vi "Parse State Queue Plus.vi"(0 "State Queue":string, 1 "Name(\"\" to use uuid)":string, 7 "Error In (no error)":errorcluster, 9 "Dequeue Timeout(0ms)":i32, 11 "Response Timeout(1000ms)":i32=1000) -> (4 "Remaining States":string, 6 "Current State":string, 8 "Arguments":string, 15 "From Who":string)   [LabVIEW 2020, in "JKI-State-Machine-Plus.lvlib"]
doc: "Parses the JKI State Machine state queue and returns the current state that will execute next with the associated arguments.\n\nFor instructions on how to use the JKI State Machine, examples and video tutorials, visit:\nhttp://jkisoft.com/state-machine/\n\n<B>Inputs:</B>\n <B>State Queue:</B> The entire state queue is wired to this input. This should come from the main JKI State Machine shift register.\n <B>Error In</B> The error cluster from the JKI State Machine is wired to this input. If an error occures and appears on this input, the current state output returns the \"Error Handler\" state.\n\n<B>Outputs:</B>\n <B>Remaining States:</B> Returns all the next states that should execute after the current state completes. These should be passed through the current state in the state machine. These can also be modified or augmented within the current state if necessary.\n <B>Current State:</B> Returns the current state that should execute next in the state machine. If an error is wired to the Error input then the current state output becomes \"Error Handler\".\n <B>Arguments:</B> Returns any argument(s) that may be used in the current state string. These arguments come after the \">>\" characters. <B>Note:</B> The arguments variable must not contain any unprintable characters like linefeed or carriage return.\n\n<B>State Syntax:</B>\nStateCategory: State >> Argument\nLine Terminator: Line feed\n <B>Example:</B>\nUI: Help >> About\n\nWhere \"UI\" is the state category\nWhere \"Help\" is the state\nWhere \"About\" is the argument\n <B>Other Examples:</B>\nApp Data: Initialize\nUI: Initialize\nHelp >> About\n\n<B>Commenting:</B>\nTo add a comment use \"//\" or \"#\" and all text to the right will be ignored\n <B>Commenting Example:</B>\nUI: Initialize // This initializes the UI\n# This whole line is a comment\n// Another comment line\n\nJKI State Machine™ 2018.0.7.45\nhttp://jki.net/state-machine/\nCopyright (C) 2005-2018, JKI <info@jki.net>\nALL RIGHTS RESERVED"
uses:
  JKI-State-Machine-Plus.lvlib
  _Cross JKI StateMachine State Data.ctl
  _Cross JKI StateMachine State Response.ctl
  _uuid.vi
  _JKISMQFGV.vi
  <vilib>/regexp/Match Regular Expression.xnode
panel:
  # "For instructions on how to use the JKI State Machine, examples and video tutorials, visit:\nhttp://jki.net/state-machine/\n\nJKI State Machine™\nhttp://jki.net/state-machine/\nCopyright (C) 2005-2017, JKI <info@jki.net>\nALL RIGHTS RESERVED"
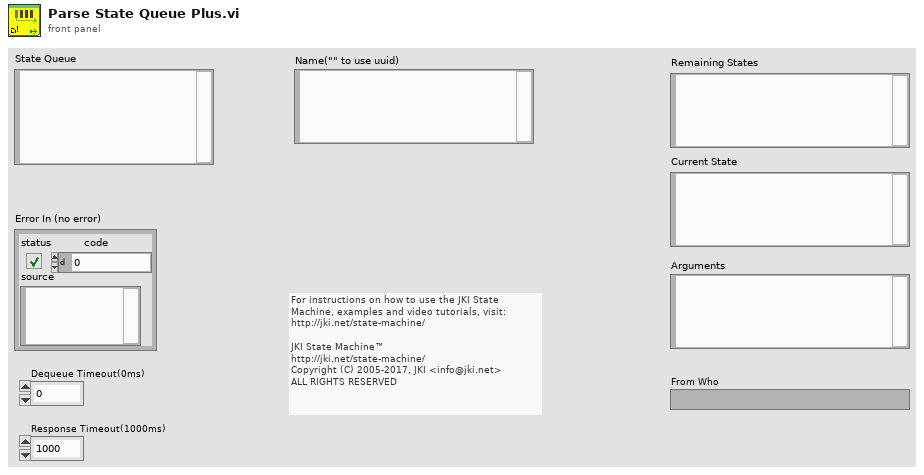
[diagram p1: front panel]
types:
  T1 = typedef "JKI-State-Machine-Plus.lvlib/_Cross JKI StateMachine State Data.ctl" = cluster{"state":string, "args":string, "source":string, "RespQ":refnum<queue>}
  T2 = typedef "JKI-State-Machine-Plus.lvlib/_Cross JKI StateMachine State Response.ctl" = cluster{"error":errorcluster}
  T3 = typedef "JKI-State-Machine-Plus.lvlib/_JKISMQ.ctl" = cluster{"Queue":refnum<queue>, "Locked Status":refnum<data-value>, "Stand Alone Mode":bool}
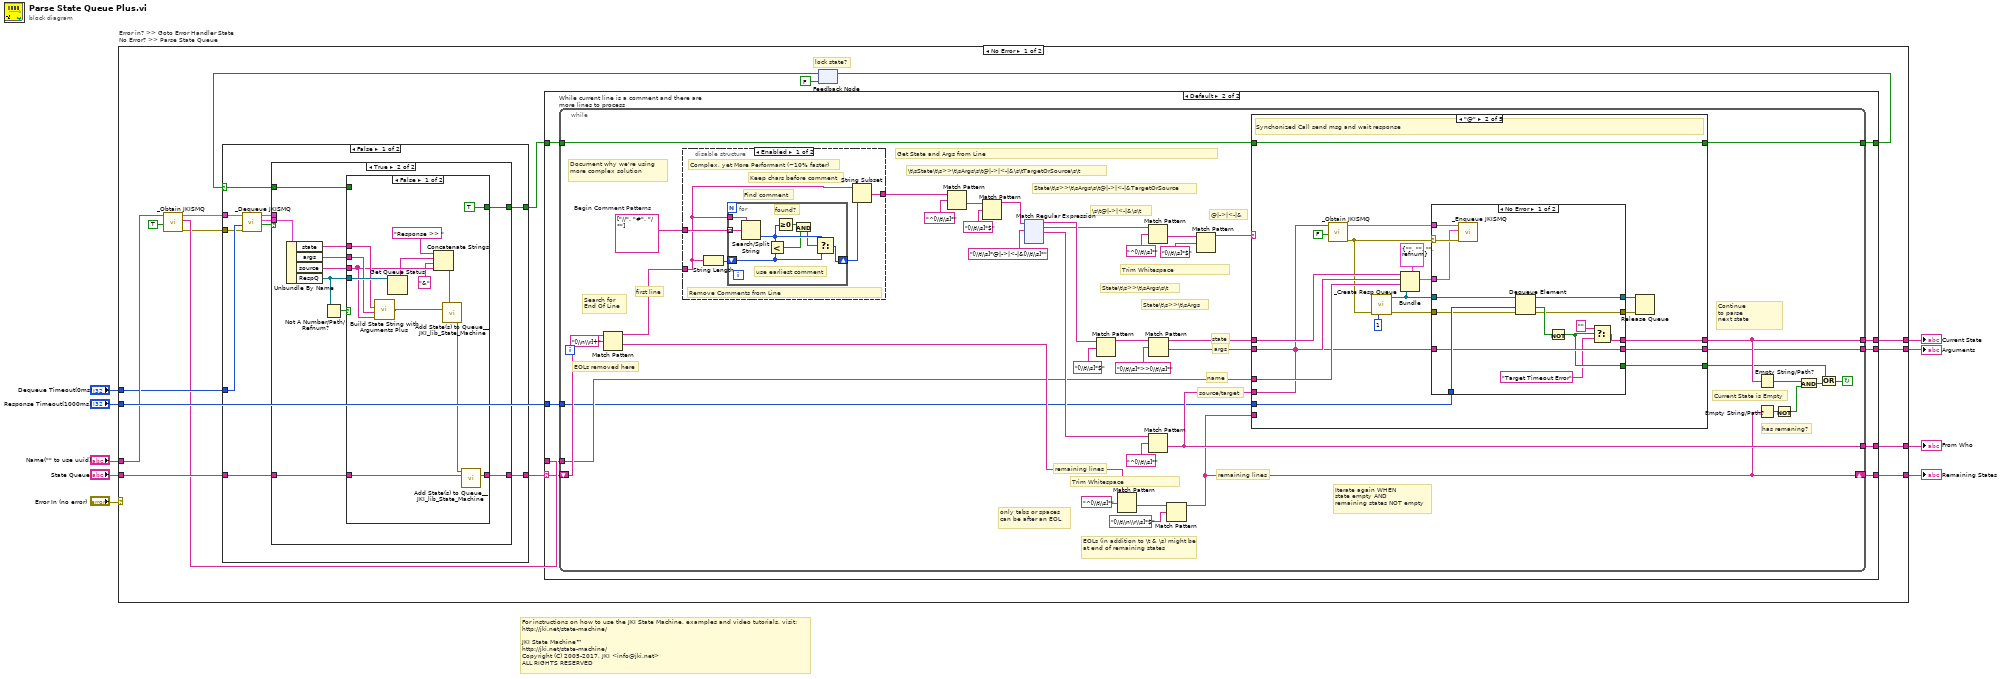
[diagram p0: block diagram]
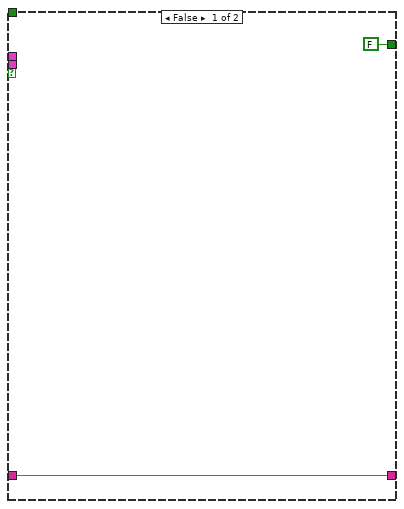
[diagram p2: hidden frame]
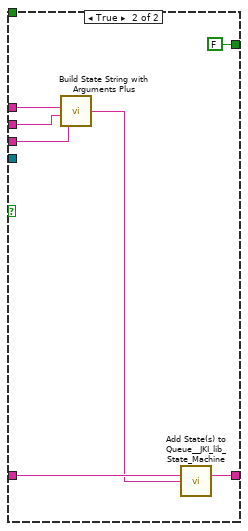
[diagram p3: hidden frame]
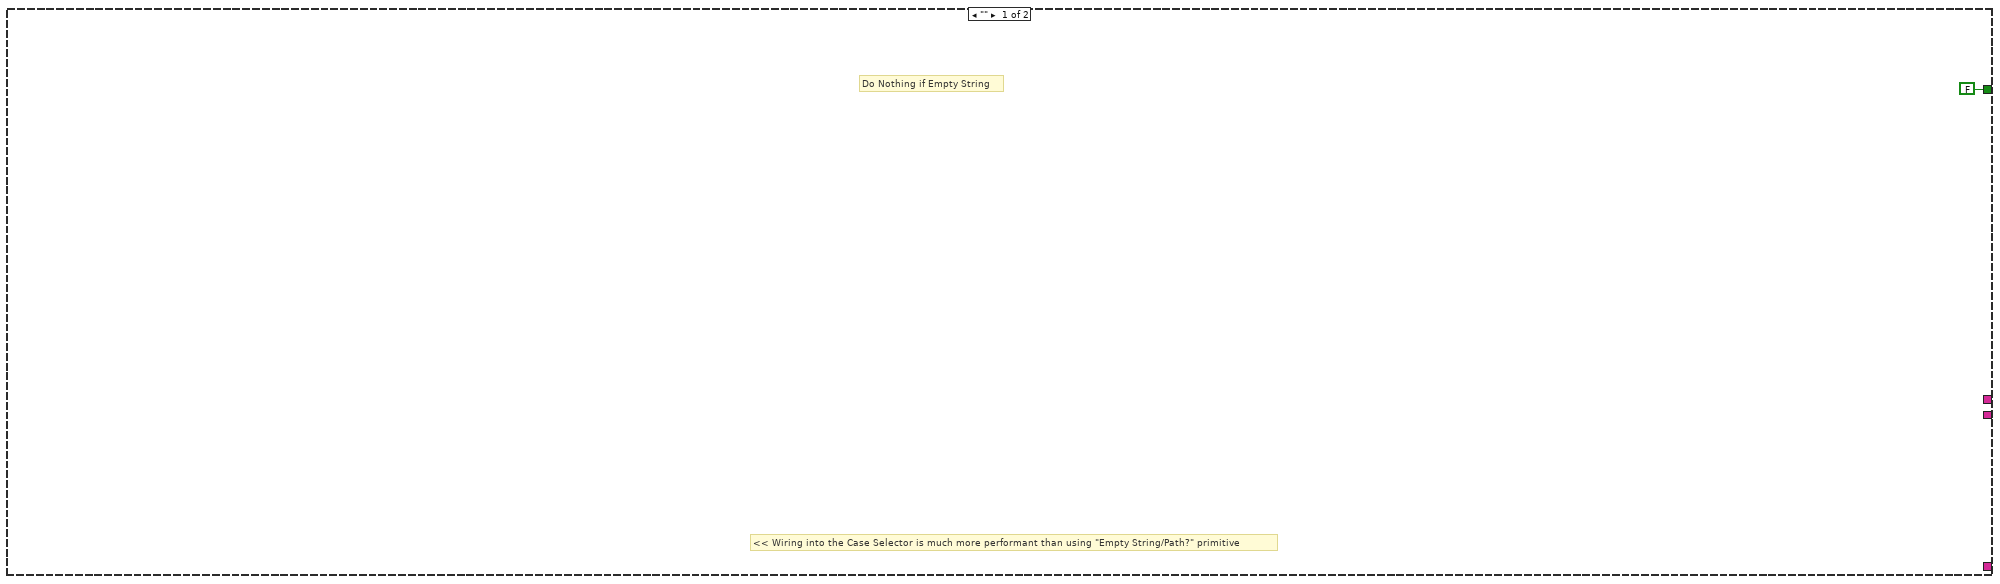
[diagram p5: hidden frame]
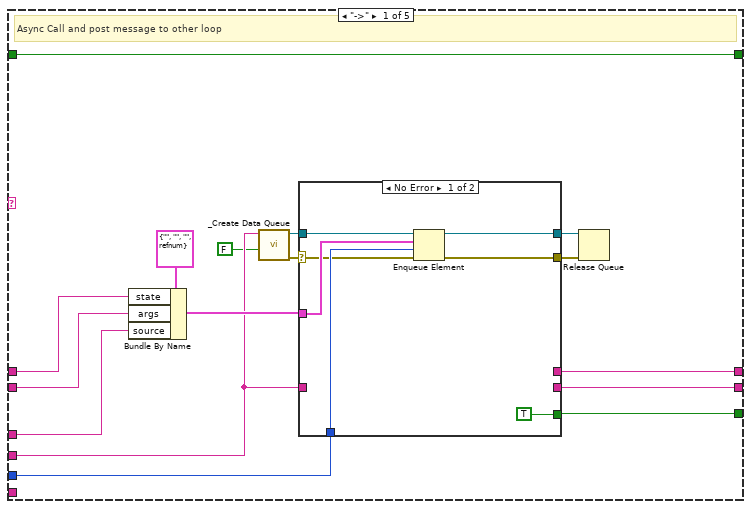
[diagram p6: hidden frame]
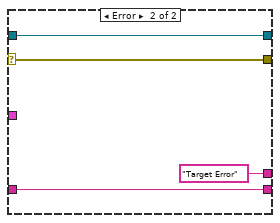
[diagram p7: hidden frame]
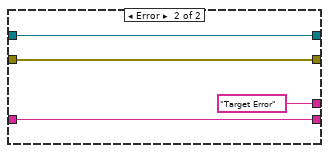
[diagram p8: hidden frame]
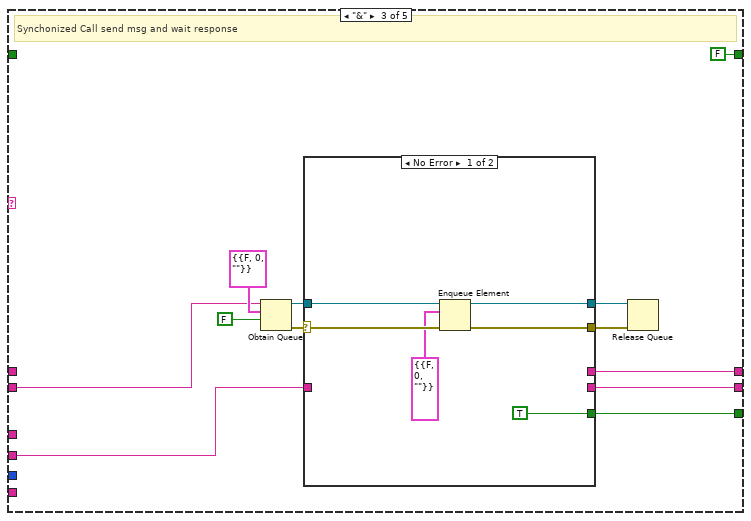
[diagram p9: hidden frame]
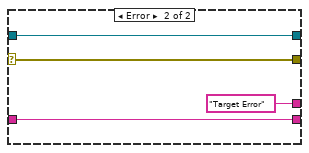
[diagram p10: hidden frame]
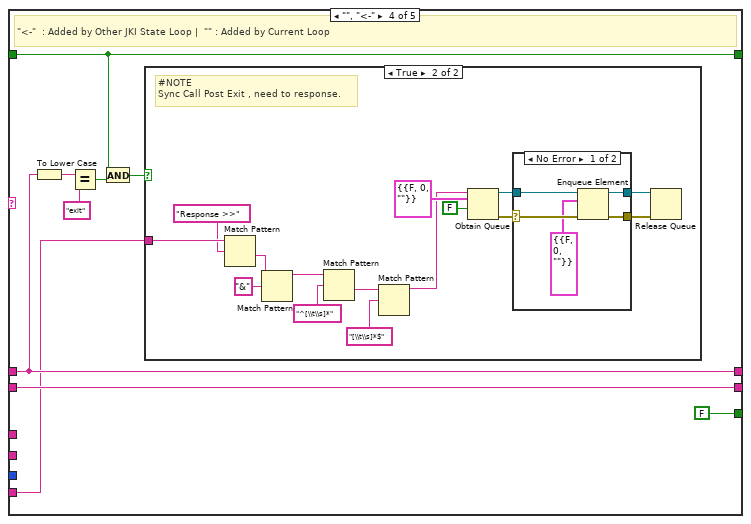
[diagram p11: hidden frame]
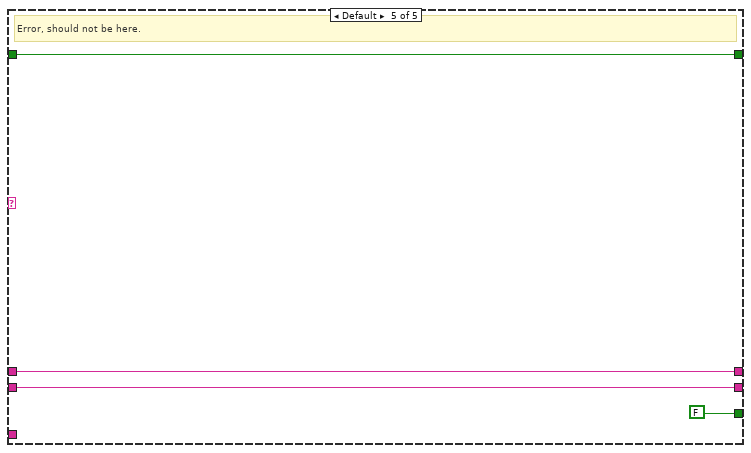
[diagram p14: hidden frame]
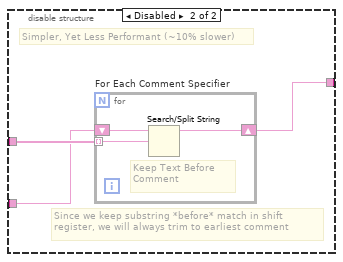
[diagram p15: hidden frame]
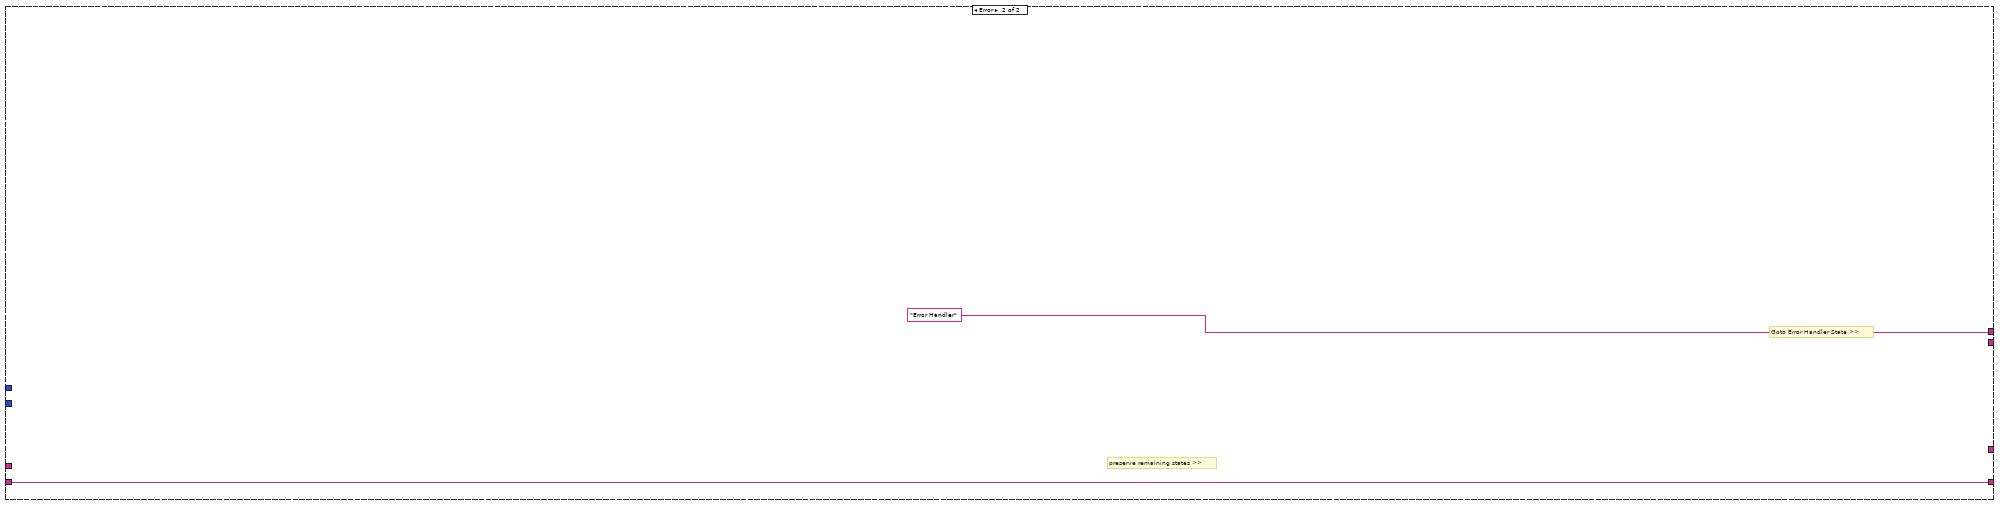
[diagram p16: hidden frame]
diagram:
  # "For instructions on how to use the JKI State Machine, examples and video tutorials, visit:\nhttp://jki.net/state-machine/\n\nJKI State Machine™\nhttp://jki.net/state-machine/\nCopyright (C) 2005-2017, JKI <info@jki.net>\nALL RIGHTS RESERVED"
  n1 = case "Error in? >> Goto Error Handler State\nNo Error? >> Parse State Queue" shown="No Error" "Error In (no error)" {
    tunnel: [w24 w377] -> w9
    tunnel: [w26 "Error Handler"] -> w7
    tunnel: [w25 _] -> w6
    tunnel: "State Queue" -> [w23 w377]
    tunnel: "Response Timeout(1000ms)" -> [w22 _]
    tunnel: "Name(\"\" to use uuid)" -> [w21 _]
    tunnel: [w20 _] -> w2
    tunnel: "Dequeue Timeout(0ms)" -> [w18 _]
    frame No Error {
      # "lock state?"
      n2 = call "_Obtain JKISMQ.vi"("create if not found? (T)"=TRUE, "Name(\"\" to use uuid) in"=w21) -> ("Error out"=w10:errorcluster, "Name"=w12:string, "JKISMQ"=w13:T3)  [unwired: 6 in, 1 out]
      n3 = feedback #1(FALSE) -> (w16:bool)
      n4 = case shown="False" w16 {
        selector: w16 -> [w34 w70]
        tunnel: w23 -> [w36 w69]
        tunnel: [w35 w69] -> w19
        tunnel: w18 -> [w31 _]
        tunnel: [w33 w70] -> w15
        tunnel: w13 -> [w32 _]
        tunnel: w10 -> [w28 _]
        frame False {
          n5 = call "_Dequeue JKISMQ.vi"("Error in"=w28, "Dequeue Timeout(0ms)"=w31, "JKISMQ"=w32) -> ("Valid?"=w30:bool, "Data"=w29:T1, "JKISMQ"=w27:T3)  [unwired: 5 in, 1 out]
          n6 = case shown="True" w30 {
            tunnel: w29 -> [_ w48]
            tunnel: w36 -> [w38 w46]
            tunnel: [w38 w45] -> w35
            tunnel: w34 -> [_ w40]
            tunnel: [FALSE w39] -> w33
            tunnel: w27 -> [_ _]
            frame False {
            }
            frame True {
              n7 = Unbundle By Name(w48) -> ("state"=w43:string, "args"=w42:string, "source"=w41:string, "RespQ"=w44:refnum<queue>)
              n8 = Not A Number/Path/Refnum?(number/path/refnum=w44) -> (NaN/Path/Refnum?=w47:bool)
              n9 = case shown="False" w47 {
                tunnel: w46 -> [w61 w68]
                tunnel: [w60 w67] -> w45
                tunnel: w44 -> [w59 _]
                tunnel: w43 -> [w54 w65]
                tunnel: w42 -> [w53 w64]
                tunnel: w41 -> [w52 w63]
                tunnel: w40 -> [_ _]
                tunnel: [TRUE FALSE] -> w39
                frame False {
                  n10 = call "Build State String with Arguments Plus.vi"("Source (\"\")"=w52, "Arguments (\"\")"=w53, "State"=w54) -> ("State with Arguments"=w55:string)  [unwired: 3 in]
                  n11 = Get Queue Status(queue=w59) -> (queue name=w51:string)  [unwired: 2 in, 7 out]
                  n12 = Concatenate Strings("Response >> " ("State(s) at Back (\"\")"), w51, "&" ("string"), w52) -> (w56:string)
                  n13 = call <vilib>:"Add State(s) to Queue__JKI_lib_State_Machine.vi"("State(s) in (\"\")"=w55, "State(s) at Back (\"\")"=w56) -> ("States Out"=w58:string)  [unwired: 13 in]
                  n14 = call <vilib>:"Add State(s) to Queue__JKI_lib_State_Machine.vi"("State(s) in Front (\"\")"=w58, "State(s) in (\"\")"=w61) -> ("States Out"=w60:string)  [unwired: 13 in]
                }
                frame True {
                  n15 = call "Build State String with Arguments Plus.vi"("Source (\"\")"=w63, "Arguments (\"\")"=w64, "State"=w65) -> ("State with Arguments"=w66:string)  [unwired: 3 in]
                  n16 = call <vilib>:"Add State(s) to Queue__JKI_lib_State_Machine.vi"("State(s) in (\"\")"=w68, "State(s) at Back (\"\")"=w66) -> ("States Out"=w67:string)  [unwired: 13 in]
                }
              }
            }
          }
        }
        frame True {
        }
      }
      n17 = case shown="Default" w19 {
        selector: w19 -> [_ w74]
        tunnel: [_ w80] -> w26
        tunnel: [_ w79] -> w25
        tunnel: [_ w78] -> w24
        tunnel: w22 -> [_ w77]
        tunnel: [_ w76] -> w20
        tunnel: w12 -> [_ w75]
        tunnel: w15 -> [_ w73]
        tunnel: [FALSE w72] -> w14
        frame "" {
          # "Do Nothing if Empty String"
          # "<< Wiring into the Case Selector is much more performant than using \"Empty String/Path?\" primitive"
        }
        frame Default {
          n18 = while "While current line is a comment and there are more lines to process" {
            tunnel: [w92] -> w80
            tunnel: [w91] -> w79
            shift-right: [w81] -> w78
            shift-left: w74 -> [w118]
            tunnel: w77 -> [w85]
            tunnel: w75 -> [w90]
            tunnel: [w89] -> w76
            tunnel: w73 -> [w83]
            tunnel: [w82] -> w72
            stop <- w88 continue-if-true
            w117 = string[] ["//", "#", "/*"]  # Begin Comment Patterns
            # "Continue\nto parse \nnext state"
            # "source/target"
            # "name"
            # "@|->|<-|&"
            # "\\s\\t@|->|<-|&\\s\\t"
            # "Trim Whitespace"
            # "State\\t\\s>>\\t\\sArgs"
            # "State\\t\\s>>\\t\\sArgs\\s\\t"
            # "Get State and Args from Line"
            # "State\\t\\s>>\\t\\sArgs\\s\\t@|->|<-|&TargetOrSource"
            # "\\t\\sState\\t\\s>>\\t\\sArgs\\s\\t@|->|<-|&\\s\\tTargetOrSource\\s\\t"
            # "remaining lines"
            # "EOLs (in addition to \\t & \\s) might be at end of remaining states"
            # "Document why we're using more complex solution"
            # "Trim Whitespace"
            # "EOLs removed here"
            # "only tabs or spaces can be after an EOL"
            # "Current State is Empty"
            # "has remaning?"
            # "remaining lines"
            # "first line"
            # "Search for End Of Line"
            # "Iterate again WHEN\nstate empty AND\nremaining states NOT empty"
            # "args"
            # "state"
            n19 = Match Pattern(string=w118, regular expression="[\\n\\r]+") -> (before substring=w115:string, after substring=w108:string)  [unwired: 1 in, 2 out]
            n20 = disable-structure "Diagram Disable Structure" shown="Enabled" {
              disable-tunnel: w117 -> [w361 w372]
              disable-tunnel: [w360 w371] -> w116
              disable-tunnel: w115 -> [w359 w370]
              frame Enabled {
                # "Remove Comments from Line"
                # "Complex, yet More Performant (~10% faster)"
                # "Keep chars before comment"
                # "Find comment"
                n21 = String Length(string=w359) -> (length=w358:i32)
                n22 = for {
                  tunnel: w361 -> [w366] mode=indexing
                  shift-right: [w368] -> w357
                  shift-left: w358 -> [w369]
                  tunnel: w359 -> [w367]
                  # "found?"
                  # "use earliest comment"
                  n23 = Search/Split String(string=w367, search string/char (-)=w366) -> (offset of match=w365:i32)  [unwired: 1 in, 2 out]
                  n24 = Less?(x=w365, y=w369) -> (x < y?=w363:bool)
                  n25 = Greater Or Equal To 0?(x=w365) -> (x >= 0?=w364:bool)
                  n26 = And(x=w364, y=w363) -> (x .and. y?=w362:bool)
                  n27 = Select(t=w365, s=w362, f=w369) -> (s? t:f=w368:i32)
                }
                n28 = String Subset(string=w359, length (rest)=w357) -> (substring=w360:string)  [unwired: 1 in]
              }
              frame Disabled {
                # "Since we keep substring *before* match in shift register, we will always trim to earliest comment"
                # "Simpler, Yet Less Performant (~10% slower)"
                n29 = for "For Each Comment Specifier" {
                  tunnel: w372 -> [w374] mode=indexing
                  shift-right: [w373] -> w371
                  shift-left: w370 -> [w375]
                  # "Keep Text Before Comment"
                  n30 = Search/Split String(string=w375, search string/char (-)=w374) -> (substring before match=w373:string)  [unwired: 1 in, 2 out]
                }
              }
            }
            n31 = Match Pattern(string=w116, regular expression="^[\\t\\s]*") -> (after substring=w106:string)  [unwired: 1 in, 3 out]
            n32 = Match Pattern(string=w106, regular expression="[\\t\\s]*$") -> (before substring=w84:string)  [unwired: 1 in, 3 out]
            n33 = xnode "Match Regular Expression"("input string"=w84, "regular expression"="[\\t\\s]*@|->|<-|&[\\t\\s]*") -> ("before match"=w103:string, "whole match"=w100:string, "after match"=w93:string)  [unwired: 4 in, 2 out]
            n34 = Match Pattern(string=w103, regular expression="[\\t\\s]*$") -> (before substring=w102:string)  [unwired: 1 in, 3 out]
            n35 = Match Pattern(string=w108, regular expression="^[\\t\\s]*") -> (after substring=w107:string)  [unwired: 1 in, 3 out]
            n36 = Match Pattern(string=w100, regular expression="^[\\t\\s]*") -> (after substring=w96:string)  [unwired: 1 in, 3 out]
            n37 = Match Pattern(string=w93, regular expression="^[\\t\\s]*") -> (after substring=w89:string)  [unwired: 1 in, 3 out]
            n38 = Match Pattern(string=w102, regular expression="[\\t\\s]*>>[\\t\\s]*") -> (before substring=w99:string, after substring=w98:string)  [unwired: 1 in, 2 out]
            n39 = Match Pattern(string=w107, regular expression="[\\t\\n\\r\\s]*$") -> (before substring=w81:string)  [unwired: 1 in, 3 out]
            n40 = Match Pattern(string=w96, regular expression="[\\t\\s]*$") -> (before substring=w95:string)  [unwired: 1 in, 3 out]
            n41 = case shown="\"@\"" w95 {
              tunnel: w99 -> [w136 w166 _ w214 w242]
              tunnel: w98 -> [w135 w165 w187 w216 w241]
              tunnel: [w128 w160 w196 w214 w242] -> w92
              tunnel: [w127 w159 w195 w216 w241] -> w91
              tunnel: w90 -> [w134 w164 _ _ _]
              tunnel: w89 -> [w126 w152 w188 _ _]
              tunnel: [w129 w161 w197 FALSE FALSE] -> w86
              tunnel: w85 -> [w132 w162 _ _ _]
              tunnel: w83 -> [w122 w153 _ w209 w239]
              tunnel: [w122 w153 FALSE w209 w239] -> w82
              tunnel: w81 -> [_ _ _ w208 _]
              frame "->" {
                # "Async Call and post message to other loop"
                n42 = Bundle By Name(cluster=T1 {"state"="", "args"="", "source"="", "RespQ"=refnum} ("Cross JKI State Machine State"), "state"=w136, "args"=w135, "source"=w134) -> (w133:T1)
                n43 = call "_Create Data Queue.vi"("create if not found? (T)"=FALSE, "Name"=w126) -> ("error out"=w124:errorcluster, "Queue out"=w125:refnum<queue>)  [unwired: 7 in, 1 out]
                n44 = case shown="No Error" w124 {
                  selector: w124 -> [w140 w147]
                  tunnel: w133 -> [w144 _]
                  tunnel: w132 -> [w143 _]
                  tunnel: w125 -> [w142 w148]
                  tunnel: [w141 w148] -> w131
                  tunnel: [w139 w147] -> w130
                  tunnel: [TRUE _] -> w129
                  tunnel: [_ "Target Error" ("before match")] -> w128
                  tunnel: [_ w145] -> w127
                  tunnel: w126 -> [_ w145]
                  frame No Error {
                    n45 = Enqueue Element(queue=w142, element=w144, timeout in ms (-1)=w143, error in (no error)=w140) -> (queue out=w141:refnum<queue>, error out=w139:errorcluster)  [unwired: 1 out]
                  }
                  frame Error {
                  }
                }
                n46 = Release Queue(queue=w131, error in (no error)=w130) -> ()  [unwired: 1 in, 3 out]
              }
              frame "@" {
                # "Synchonized Call send msg and wait response"
                n47 = call "_Obtain JKISMQ.vi"("create if not found? (T)"=FALSE, "Name(\"\" to use uuid) in"=w152) -> ("Error out"=w150:errorcluster, "JKISMQ"=w151:T3)  [unwired: 6 in, 2 out]
                n48 = call "_Create Resp Queue.vi"("max queue size (-1, unlimited)"=1, "error in (no error)"=w150) -> ("error out"=w155:errorcluster, "queue out"=w157:refnum<queue>)  [unwired: 7 in, 1 out]
                n49 = Bundle(cluster=T1 {"state"="", "args"="", "source"="", "RespQ"=refnum} ("Cross JKI State Machine State"), "state"=w166, "args"=w165, "source"=w164, "RespQ"=w157) -> (w163:T1)
                n50 = case shown="No Error" w150 {
                  selector: w150 -> [w180 _]
                  tunnel: w163 -> [w179 _]
                  tunnel: w162 -> [w178 _]
                  tunnel: w151 -> [w181 _]
                  tunnel: [w174 _] -> w161
                  tunnel: [w177 "Target Error" ("before match")] -> w160
                  tunnel: [w176 w184] -> w159
                  tunnel: w152 -> [w176 w184]
                  tunnel: w157 -> [w171 w183]
                  tunnel: [w170 w183] -> w156
                  tunnel: w155 -> [w169 w182]
                  tunnel: [w168 w182] -> w154
                  frame No Error {
                    n51 = call "_Enqueue JKISMQ.vi"("Error in"=w180, "Data"=w179, "JKISMQ"=w181) -> ()  [unwired: 7 in, 2 out]
                    n52 = Dequeue Element(queue=w171, timeout in ms (-1)=w178, error in (no error)=w169) -> (queue out=w170:refnum<queue>, timed out?=w175:bool, error out=w168:errorcluster)  [unwired: 1 out]
                    n53 = Not(x=w175) -> (.not. x?=w174:bool)
                    n54 = Select(t="" ("f"), s=w174, f="Target Timeout Error" ("before match")) -> (s? t:f=w177:string)
                  }
                  frame Error {
                  }
                }
                n55 = Release Queue(queue=w156, error in (no error)=w154) -> ()  [unwired: 1 in, 3 out]
              }
              frame "&" {
                # "Synchonized Call send msg and wait response"
                n56 = Obtain Queue(name (unnamed)=w187, element data type=T2 {"error"={"status"=FALSE, "code"=0, "source"=""}} ("Cross JKI State Machine Response"), create if not found? (T)=FALSE) -> (queue out=w192:refnum<queue>, error out=w191:errorcluster)  [unwired: 2 in, 1 out]
                n57 = case shown="No Error" w191 {
                  selector: w191 -> [w201 w205]
                  tunnel: [TRUE _] -> w197
                  tunnel: [_ "Target Error" ("before match")] -> w196
                  tunnel: [_ w204] -> w195
                  tunnel: w192 -> [w203 w206]
                  tunnel: [w202 w206] -> w194
                  tunnel: [w200 w205] -> w193
                  tunnel: w188 -> [_ w204]
                  frame No Error {
                    n58 = Enqueue Element(queue=w203, element=T2 {"error"={"status"=FALSE, "code"=0, "source"=""}}, error in (no error)=w201) -> (queue out=w202:refnum<queue>, error out=w200:errorcluster)  [unwired: 1 in, 1 out]
                  }
                  frame Error {
                  }
                }
                n59 = Release Queue(queue=w194, error in (no error)=w193) -> ()  [unwired: 1 in, 3 out]
              }
              frame "", "<-" {
                # "\"<-\"  : Added by Other JKI State Loop |  \"\" : Added by Current Loop"
                n60 = To Lower Case(string=w214) -> (all lower case string=w213:string)
                n61 = Equal?(x=w213, y="exit") -> (x = y?=w210:bool)
                n62 = And(x=w209, y=w210) -> (x .and. y?=w211:bool)
                n63 = case shown="True" w211 {
                  tunnel: w208 -> [_ w225]
                  frame False {
                  }
                  frame True {
                    # "#NOTE\nSync Call Post Exit , need to response."
                    n64 = Match Pattern(string=w225, regular expression="Response >>") -> (after substring=w222:string)  [unwired: 1 in, 3 out]
                    n65 = Match Pattern(string=w222, regular expression="&") -> (before substring=w218:string)  [unwired: 1 in, 3 out]
                    n66 = Match Pattern(string=w218, regular expression="^[\\t\\s]*") -> (after substring=w221:string)  [unwired: 1 in, 3 out]
                    n67 = Match Pattern(string=w221, regular expression="[\\t\\s]*$") -> (before substring=w217:string)  [unwired: 1 in, 3 out]
                    n68 = Obtain Queue(name (unnamed)=w217, element data type=T2 {"error"={"status"=FALSE, "code"=0, "source"=""}} ("Cross JKI State Machine Response"), create if not found? (T)=FALSE) -> (queue out=w230:refnum<queue>, error out=w231:errorcluster)  [unwired: 2 in, 1 out]
                    n69 = case shown="No Error" w231 {
                      selector: w231 -> [w234 w237]
                      tunnel: w230 -> [w236 w238]
                      tunnel: [w235 w238] -> w228
                      tunnel: [w233 w237] -> w229
                      frame No Error {
                        n70 = Enqueue Element(queue=w236, element=T2 {"error"={"status"=FALSE, "code"=0, "source"=""}}, error in (no error)=w234) -> (queue out=w235:refnum<queue>, error out=w233:errorcluster)  [unwired: 1 in, 1 out]
                      }
                      frame Error {
                      }
                    }
                    n71 = Release Queue(queue=w228, error in (no error)=w229) -> ()  [unwired: 1 in, 3 out]
                  }
                }
              }
              frame Default {
                # "Error, should not be here."
              }
            }
            n72 = Empty String/Path?(string/path=w92) -> (empty?=w121:bool)
            n73 = Empty String/Path?(string/path=w81) -> (empty?=w120:bool)
            n74 = Not(x=w120) -> (.not. x?=w114:bool)
            n75 = And(x=w121, y=w114) -> (x .and. y?=w87:bool)
            n76 = Or(x=w86, y=w87) -> (x .or. y?=w88:bool)
          }
        }
      }
      n77 = feedback-in #1(w14) -> ()
    }
    frame Error {
      # "Goto Error Handler State >>"
      # "preserve remaining states >>"
    }
  }
  "Remaining States" <- w9
  "Arguments" <- w6
  "Current State" <- w7
  "From Who" <- w2
